vi "RollerDoubleSolenoid.vi"(7 "State":T4=enum."Out", 8 "Error in":errorcluster, 11 "SolenoidDevRef":T1={"DevStatus"={"status"=FALSE, "code"=0, "source"=""}, "Solenoid Module"=enum."Solenoid Module 1", "Forward Solenoid Channel"=enum."Invalid", "Reverse Solenoid Channel"=enum."Invalid"}) -> (0 "Error out":errorcluster)   [LabVIEW 2013]
uses:
  <vilib>/Rock Robotics/WPI/Solenoid/WPI_SolenoidValue.ctl
  <vilib>/Rock Robotics/WPI/Solenoid/WPI_SolenoidSetEnum.vi
  DoubleSolenoidControl.ctl
  <vilib>/Rock Robotics/WPI/Solenoid/WPI_SolenoidChannel.ctl
  <vilib>/Rock Robotics/SystemInterfaces/Typedef/FPGA_TypedefSolenoidModule.ctl
  <vilib>/Rock Robotics/WPI/Solenoid/WPI_SolenoidDevRef.ctl
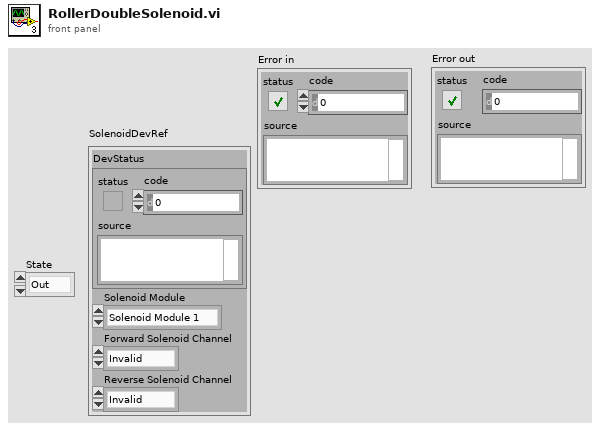
[diagram p1: front panel]
types:
  T1 = typedef "WPI_SolenoidDevRef.ctl" = cluster{"DevStatus":errorcluster, "Solenoid Module":T2, "Forward Solenoid Channel":T3, "Reverse Solenoid Channel":T3}
  T2 = typedef "FPGA_TypedefSolenoidModule.ctl" = enum16{"Solenoid Module 1", "Solenoid Module 2"}
  T3 = typedef "WPI_SolenoidChannel.ctl" = enum8{"Solenoid 1", "Solenoid 2", "Solenoid 3", "Solenoid 4", "Solenoid 5", "Solenoid 6", "Solenoid 7", "Solenoid 8", "Invalid"}
  T4 = typedef "DoubleSolenoidControl.ctl" = enum16{"Init", "Out", "In", "Middle"}
  T5 = typedef "WPI_SolenoidValue.ctl" = enum16{"Off", "On", "Forward", "Reverse"}
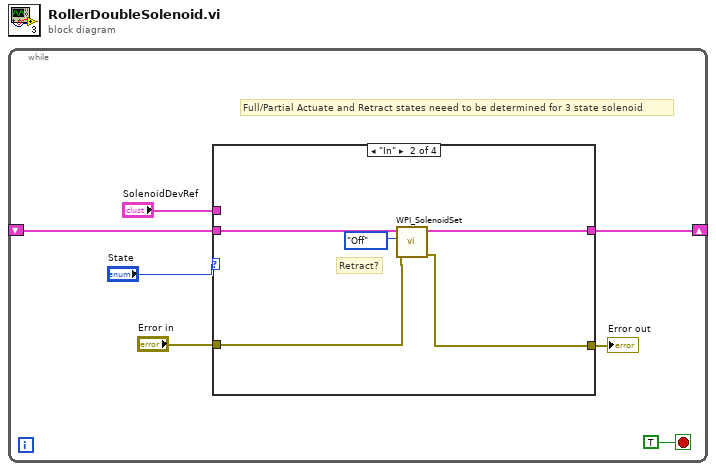
[diagram p0: block diagram]
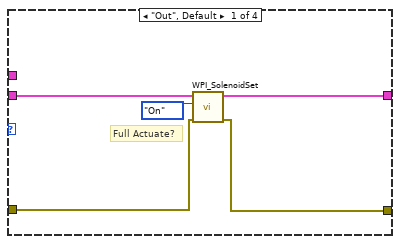
[diagram p2: hidden frame]
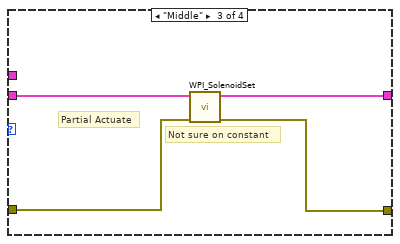
[diagram p3: hidden frame]
diagram:
  n1 = while {
    shift-right: [w4] -> _
    shift-left: _ -> [w6]
    stop <- TRUE stop-if-true
    # "Full/Partial Actuate and Retract states neeed to be determined for 3 state solenoid"
    n2 = case shown="\"In\"" "State" {
      tunnel: [w11 w16 w21 w23] -> w4
      tunnel: w6 -> [w12 w17 w20 _]
      tunnel: "SolenoidDevRef" -> [_ _ _ w23]
      tunnel: [w8 w13 w18 w22] -> w1
      tunnel: "Error in" -> [w9 w14 w19 w22]
      frame "Out", Default {
        # "Full Actuate?"
        n3 = call-poly <vilib>:"WPI_SolenoidSet.vi"("error in (no error)"=w9, "Value"=WPI_SolenoidValue."On", "SolenoidDevRef"=w12) -> ("error out"=w8:errorcluster, "SolenoidDevRef"=w11:T1)  [unwired: 7 in]
      }
      frame "In" {
        # "Retract?"
        n4 = call-poly <vilib>:"WPI_SolenoidSet.vi"("error in (no error)"=w14, "Value"=WPI_SolenoidValue."Off", "SolenoidDevRef"=w17) -> ("error out"=w13:errorcluster, "SolenoidDevRef"=w16:T1)  [unwired: 7 in]
      }
      frame "Middle" {
        # "Not sure on constant"
        # "Partial Actuate"
        n5 = call-poly <vilib>:"WPI_SolenoidSet.vi"("error in (no error)"=w19, "SolenoidDevRef"=w20) -> ("error out"=w18:errorcluster, "SolenoidDevRef"=w21:T1)  [unwired: 8 in]
      }
      frame "Init" {
      }
    }
    "Error out" <- w1
  }
